vi "disable driver after move.vi"(4 "channel number":string, 5 "Msg in":T1, 6 "channel index":i32, 7 "Numeric":i32, 8 "error in (no error)":errorcluster, 9 "Device and Axis":string, 10 "VISA resource name in":refnum<visa-resource-name>, 11 "ZaberASeries in":refnum<class "ZaberASeries.lvclass">) -> (0 "error out":errorcluster, 2 "VISA resource name out":refnum<visa-resource-name>, 3 "ZaberASeries out":refnum<class "ZaberASeries.lvclass">)   [LabVIEW 2020, in "ZaberASeries.lvclass"]
uses:
  ZaberASeries.lvclass
  DriverMsg.ctl
  ZaberASeries.lvclass/ZaberASeries.ctl
  OnOffTypeDef.ctl
  Zaber A Series.lvlib
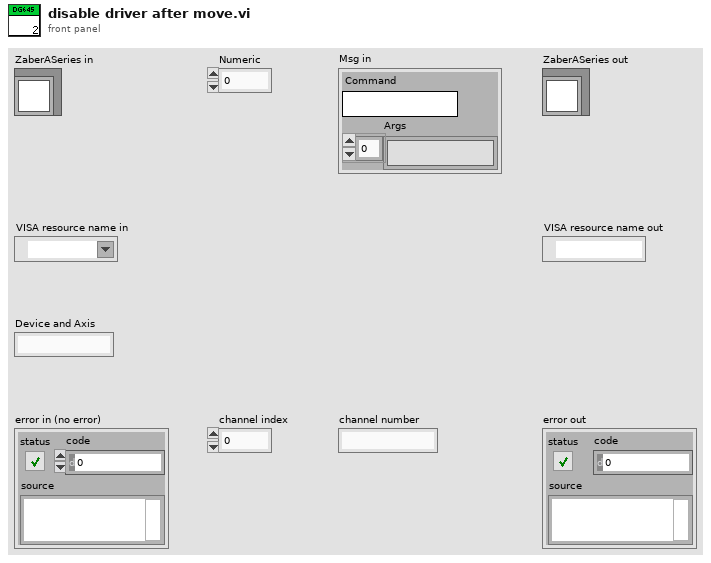
[diagram p1: front panel]
types:
  T1 = typedef "DriverMsg.ctl" = cluster{"Command":string, "Args":string[]}
  T2 = typedef "OnOffTypeDef.ctl" = enum16{"off", "on"}
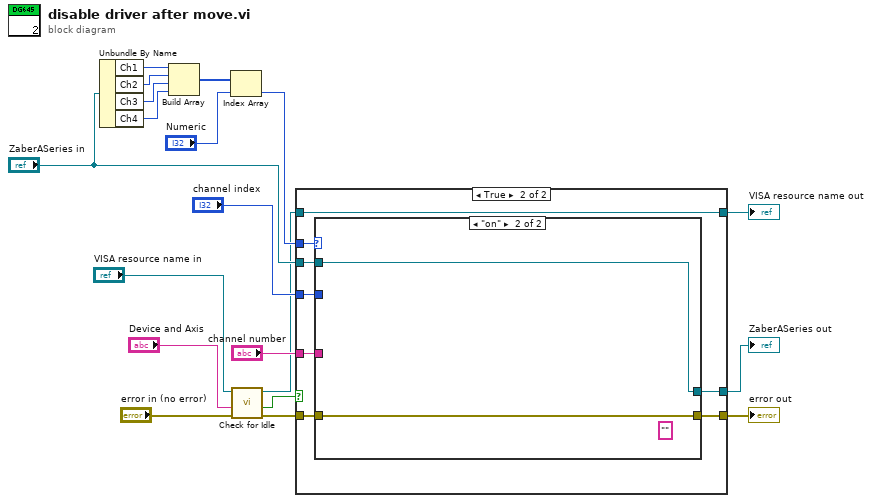
[diagram p0: block diagram]
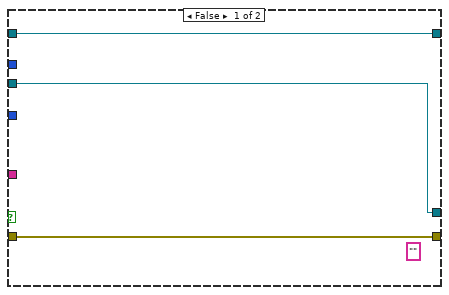
[diagram p2: hidden frame]
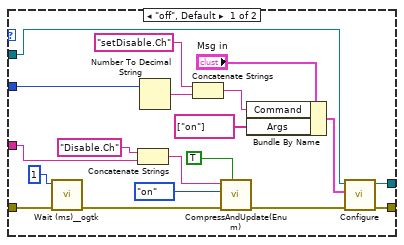
[diagram p3: hidden frame]
diagram:
  n1 = Unbundle By Name("ZaberASeries in") -> ("Ch1"=w14:T2, "Ch2"=w13:T2, "Ch3"=w12:T2, "Ch4"=w11:T2)
  n2 = Build Array(w14, w13, w12, w11) -> (w10:T2[])
  n3 = Index Array(array=w10, index="Numeric") -> (element=w17:T2)
  n4 = call "Check for Idle.vi"("error in (no error)"="error in (no error)", "Device and Axis"="Device and Axis", "VISA resource name"="VISA resource name in") -> ("error out"=w15:errorcluster, "Idle"=w9:bool, "VISA resource name out"=w6:refnum<visa-resource-name>)  [unwired: 6 in]
  n5 = case shown="True" w9 {
    tunnel: w15 -> [w22 w27]
    tunnel: [w22 w29] -> w4
    tunnel: [w21 w30] -> w5
    tunnel: w6 -> [w21 w30]
    tunnel: "channel index" -> [_ w28]
    tunnel: w17 -> [_ w26]
    tunnel: "channel number" -> [_ w25]
    tunnel: "ZaberASeries in" -> [w20 w24]
    tunnel: [w20 w23] -> w19
    frame False {
      (unwired) "" ("new commands")
    }
    frame True {
      n6 = case shown="\"on\"" w26 {
        tunnel: [w38 w51] -> w29
        tunnel: w28 -> [w47 _]
        tunnel: w27 -> [w46 w51]
        tunnel: w25 -> [w42 _]
        tunnel: w24 -> [w37 w50]
        tunnel: [w36 w50] -> w23
        frame "off", Default {
          n7 = call "Wait (ms)__ogtk.vi"("error in (no error)"=w46, "milliseconds to wait"=u32 1) -> ("error out"=w40:errorcluster)  [unwired: 8 in, 1 out]
          n8 = Concatenate Strings("Disable.Ch" ("command or variable name"), w42) -> (w44:string)
          n9 = Number To Decimal String(number=w47) -> (decimal integer string=w48:string)  [unwired: 1 in]
          n10 = Concatenate Strings("setDisable.Ch" ("string"), w48) -> (w33:string)
          n11 = call "CompressAndUpdate(Enum).vi"("force CVT update (false)"=TRUE, "error in"=w40, "enum variant"=OnOffTypeDef."on" ("Ch4"), "command or variable name"=w44) -> ("error out"=w39:errorcluster)  [unwired: 7 in]
          n12 = Bundle By Name(cluster="Msg in", "Command"=w33, "Args"=string[] ["on"]) -> (w32:T1)
          n13 = call-dynamic "Configure.vi"("error in (no error)"=w39, "Msg in"=w32, "ZaberASeries in"=w37) -> ("error out"=w38:errorcluster, "ZaberASeries out"=w36:refnum<class "ZaberASeries.lvclass">)  [unwired: 5 in, 2 out]
        }
        frame "on" {
          (unwired) "" ("new commands")
        }
      }
    }
  }
  "ZaberASeries out" <- w19
  "VISA resource name out" <- w5
  "error out" <- w4
